vi "PerformScan.vi"(0 "Avg Num Mod":i32=1, 1 "Therapy/AVG ?":bool, 2 "AlazarCluster":T9, 5 "Line Axis":i32=1 min=1 max=4, 7 "Type of scan":T10, 9 "lines per scan plane mod":i32=128, 11 "Reverse ?":bool, 12 "Digitizer Settings":T5={"Digitizer delay (us) "=0.0, "rf points per line"=2048, "lines per plane"=128, "Samp Rate (Hz)"=100000000.0, "Additional dig delay (us)"=0.0, "Voltage Scale"=0.4, "Pre-Looks"=0, "Offset delay (us)"=0.0, "bits A/D"=8, "Avg Num"=1, "DigTimeOut"=5.0, "Rel Dig Delay"=0.0, "Dig Ch"=0, "LeCroyCluster"={"LeCroy Channels"=[TRUE, FALSE, FALSE, FALSE], "LC read pt offset"=0.0, "Sweep Avg"=FALSE}, "Main Digitizer"=enum."NI Digitizer", "Dig Config"=enum."Single channel", "Digitizer ID Cluster"={"Acqiris/Alazar/SP ID"=[], "NI Instr Handles"=[], "LeCroy VISA"="", "GaGe Handle"={"Handle"=0, "Sample size"=0, "Resolution"=0, "Offset"=0, "Channels"=0, "Boards"=0}, "ATS Ref"="ATS9350", "Acqiris Address"=["PCI::INSTR0"], "ADQRef"=refnum, "adq_cu_ptr"=refnum}, "Trigger Settings"={"Trig Source"=1, "Trig Coupling"=0, "Trig Slope"=0, "Level (mV)"=1500.0}, "Bulk Acq"=FALSE, "Bulk Start Indexes"=[], "Data Ref RF"=refnum, "NI ID/Channel"=[], "Total Dig CH"=1, "Xtra Ann Trig delay (us)"=10.0, "Fix Z Delay?"=FALSE, "One Way Transmission?"=FALSE, "Data Ref Log"=refnum} {"Trigger Settings"."Trig Slope" items=["Positive", "Negative"]; "Trigger Settings"."Level (mV)" format="%.2f"; "Trigger Settings"."Trig Coupling" items=["DC 1 MOhm", "AC 1 MOhm", "DC 50 Ohm", "AC 50 Ohm"]; "Trigger Settings"."Trig Source" items=["Chan 1", "External"]; "Rel Dig Delay" format="%.2f"; "DigTimeOut" format="%.2f"; "Avg Num" min=1; "Offset delay (us)" format="%.2f"; "Additional dig delay (us)" format="%.2f"; "Digitizer delay (us)" format="%.2f"}, 13 "Motion Settings In":T1={"No Motion?"=FALSE, "Motion System"=enum."NI 735x", "Motion Bd ID"=1, "Motion Profile"="SMAC1", "# Axis"=1, "Reverse Z axis?"=TRUE, "SMAC Axis"=0, "scan pair"=enum."y-(x) scan", "RT fps"=6.0, "Steps per mm"=[1000, 1000, 1000, 1000], "Motor Parameters"={"velocity ct/s"=[10000.0, 10000.0, 10000.0, 50000.0], "accel ct/s^2"=[50000.0, 50000.0, 50000.0, 200000.0]}, "One Way Scan"=FALSE, "Reverse One Way Scan"=FALSE, "Global Position (mm)"=[], "Plane"=0, "Distance between\nscan lines (um)"=0.0, "Distance between\nscan planes (um)"=0.0, "number of scan planes"=1, "Total steps in line"=0, "Xtra plane\ndistance  (um)"=100, "Xtra planes "=1, "Add Axis"=FALSE, "overshoot cts"=200, "BKPT Shift"=0, "Scan Start Time (ms)"=0, "ESP VISA"="GPIB::1::INSTR", "3rd Axis"=1, "GL Ref Out"=refnum, "Galil Address"=""} {"3rd Axis" items=["x", "y", "z", "w"]; "Xtra planes" min=1; "Xtra plane\ndistance  (um)" min=0; "Distance between\nscan planes (um)" format="%.2f"; "Distance between\nscan lines (um)" format="%.2f"; "SMAC Axis" items=["None"=0, "Axis 1"=1, "Axis 2"=2, "Axis 3"=3, "Axis 4"=4, "Axis 5"=5, "Axis 6"=6, "Axis 7"=7, "Axis 8"=8, "Vector Space 1"=17, "Vector Space 2"=18, "Vector Space 3"=19, "Vector Space 4"=20]; "Motion Bd ID" min=1 max=32 step=1}, 14 "File Names":string[](array[string]), 15 "Offset":dbl format="%.2f") -> ()   [LabVIEW 2022 SP3]
uses:
  -ScanSystem/Controls/ScanType2.ctl
  Digitizers/-DigitizerRoutines/DigitizerSettings.ctl
  Digitizers/-DigitizerRoutines/Digitizer.ctl
  Digitizers/-DigitizerRoutines/DigConfig.ctl
  Digitizers/-DigitizerRoutines/DigitizerID.ctl
  C:/Windows/System32/ADQAPI_dotNet_helper.dll
  MotionParameters.ctl
  MotionSys.ctl
  -MotionRoutines/ScanAxis.ctl
  -MotionRoutines/3rdAxis.ctl
  Galil/Command Menu.ctl
  <vilib>/Motion/FlexMotion/CustomControls/CustomControls.llb/Program.flx
panel:
  # "allows movement down axis where pulse is sent out every time Step to Move has\nbeen moved. Small program is sent to MM2000 and executed. Motion is kind of slow."
  # "1-D and 2-D B scan settings"
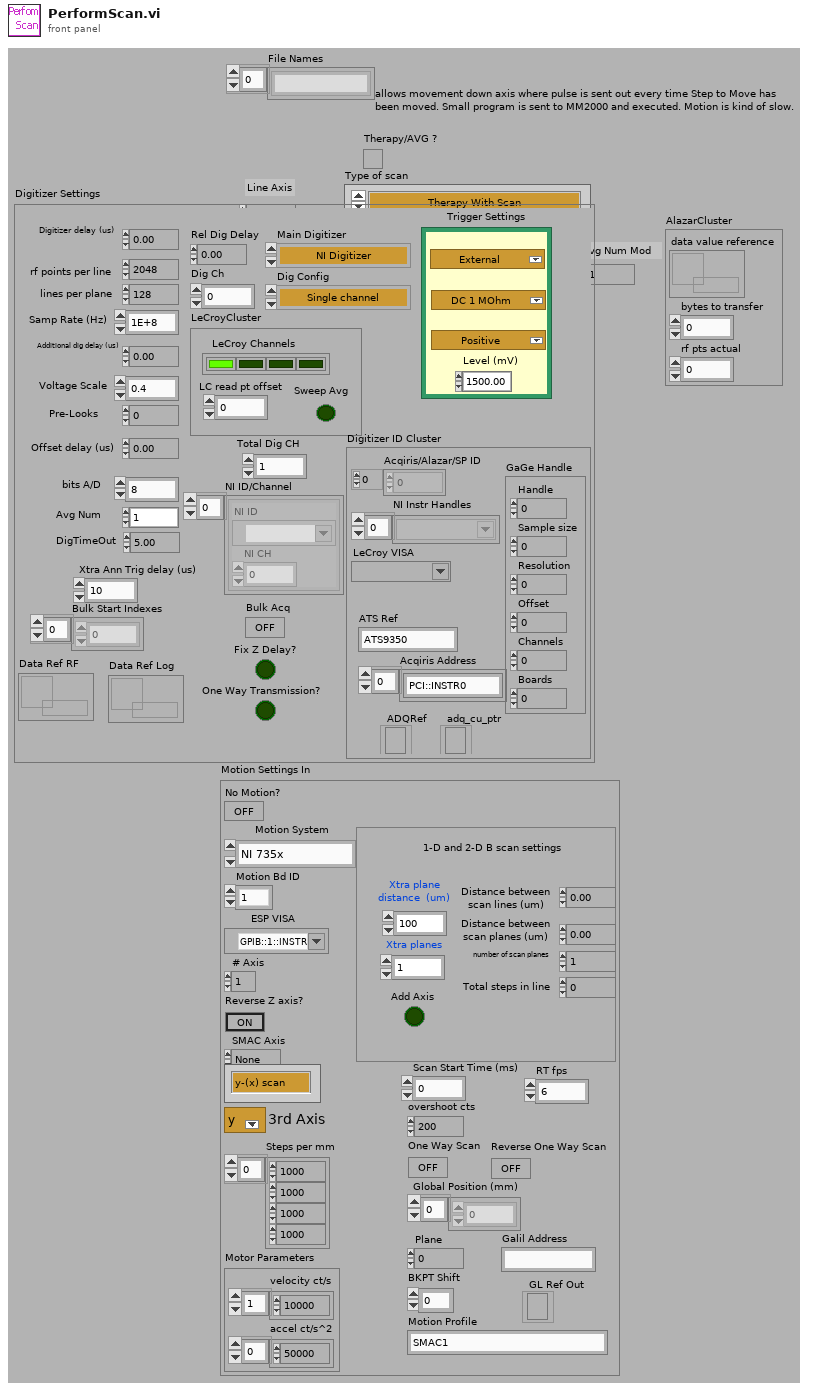
[diagram p1: front panel]
types:
  T1 = typedef "MotionParameters.ctl" = cluster{"No Motion?":bool, "Motion System":T2, "Motion Bd ID":u8, "Motion Profile":string, "# Axis":i8, "Reverse Z axis?":bool, "SMAC Axis":u16, "scan pair":T3, "RT fps":sgl, "Steps per mm":i32[], "Motor Parameters":cluster{"velocity ct/s":dbl[], "accel ct/s^2":dbl[]}, "One Way Scan":bool, "Reverse One Way Scan":bool, "Global Position (mm)":dbl[], "Plane":i32, "Distance between\nscan lines (um)":sgl, "Distance between\nscan planes (um)":sgl, "number of scan planes":i32, "Total steps in line":i32, "Xtra plane\ndistance  (um)":i32, "Xtra planes ":i32, "Add Axis":bool, "overshoot cts":i32, "BKPT Shift":i32, "Scan Start Time (ms)":u32, "ESP VISA":refnum<visa-resource-name>, "3rd Axis":T4, "GL Ref Out":refnum<k7>, "Galil Address":string}
  T2 = typedef "MotionSys.ctl" = enum16{"MM3000", "NI 735x", "Newport ESP", "No Motion Card", "Galil"}
  T3 = typedef "ScanAxis.ctl" = enum16{"y-(x) scan", "x-(y) scan", "z-(x) scan", "z-(y) scan", "y-(z) scan", "x-(z) scan", "w-(x) scan", "w-(y) scan", "w-(z) scan", "x-(w) scan", "y-(w) scan", "z-(w) scan"}
  T4 = typedef "3rdAxis.ctl" = u16
  T5 = typedef "DigitizerSettings.ctl" = cluster{"Digitizer delay (us) ":dbl, "rf points per line":i32, "lines per plane":i32, "Samp Rate (Hz)":dbl, "Additional dig delay (us)":dbl, "Voltage Scale":dbl, "Pre-Looks":i32, "Offset delay (us)":dbl, "bits A/D":i8, "Avg Num":i32, "DigTimeOut":sgl, "Rel Dig Delay":sgl, "Dig Ch":i32, "LeCroyCluster":cluster{"LeCroy Channels":bool[], "LC read pt offset":dbl, "Sweep Avg":bool}, "Main Digitizer":T6, "Dig Config":T7, "Digitizer ID Cluster":T8, "Trigger Settings":cluster{"Trig Source":u16, "Trig Coupling":u16, "Trig Slope":u16, "Level (mV)":dbl}, "Bulk Acq":bool, "Bulk Start Indexes":i32[], "Data Ref RF":refnum<data-value>, "NI ID/Channel":cluster{"NI ID":refnum<k15>, "NI CH":i32}[], "Total Dig CH":i32, "Xtra Ann Trig delay (us)":dbl, "Fix Z Delay?":bool, "One Way Transmission?":bool, "Data Ref Log":refnum<data-value>}
  T6 = typedef "Digitizer.ctl" = enum16{"Acqiris Digitizer", "NI Digitizer", "LeCroy", "GaGe", "AlazarTech", "No Digitizer", "Teledyne"}
  T7 = typedef "DigConfig.ctl" = enum16{"Single channel", "2 Chans w/ 2 Acqiris", "2 Chans w/ 1 Acqiris", "5-CH Pulser New", "5-CH pulser w/ ann array", "5-pass style ann array", "Empty"}
  T8 = typedef "DigitizerID.ctl" = cluster{"Acqiris/Alazar/SP ID":u32[], "NI Instr Handles":refnum<k15>[], "LeCroy VISA":refnum<visa-resource-name>, "GaGe Handle":cluster{"Handle":u32, "Sample size":u32, "Resolution":i32, "Offset":i32, "Channels":u32, "Boards":u32}, "ATS Ref":string, "Acqiris Address":string[], "ADQRef":refnum<k24>, "adq_cu_ptr":refnum<k24>}
  T9 = cluster{"data value reference":refnum<data-value>, "bytes to transfer":u32, "rf pts actual":u32}
  T10 = typedef "ScanType2.ctl" = enum16{"Therapy With Scan", "M scan", "M Scan With Therapy Burst", "1-D B Scan", "1-D B Scan With Therapy Burst", "2-D B Scan", "2-D B Scan With Therapy Burst", "Rotational Scan", "1-D B-Scan PRF", "2-D B-Scan PRF", "Real-Time Scan", "Contrast Agents", "1-D w/ Real-Time Set Up", "Dual Transducer", "Acoustic Microscopy", "Hydrophone Scanning"}
  T11 = typedef "Program.flx" = u8
  T12 = enum16{"Run/Stop", "Motor Off", "Velocity Threshold", "Move Complete"}
  T13 = typedef "Command Menu.ctl" = enum16{"CommandPassThrough", "Abort Motion", "Define Pos", "Velocity", "Acceleration", "Deceleration", "Position Rel", "Postion Abs", "Begin Move", "After Move", "Home", "KI", "KD", "KP", "IL", "Config I/O", "Set Bit", "Clear Bit", "Motor Off", "Moto On", "Status", "Execute", "Halt Execute", "HX Status", "Tell Velocity", "Check Motion", "BreakPoint", "Tell Position", "Current Code Line", "Tell Switches", "OC Force On", "OC Off", "Pos Soft Limit", "Rev Soft Limit"}
  T14 = typedef "Bd Id Out" = u8
  T15 = typedef "Resource Out (Enum).flx" = u16
  T16 = typedef "Axis Status (8 axes).flx" = cluster{"1":bool, "2":bool, "3":bool, "4":bool, "5":bool, "6":bool, "7":bool, "8":bool}
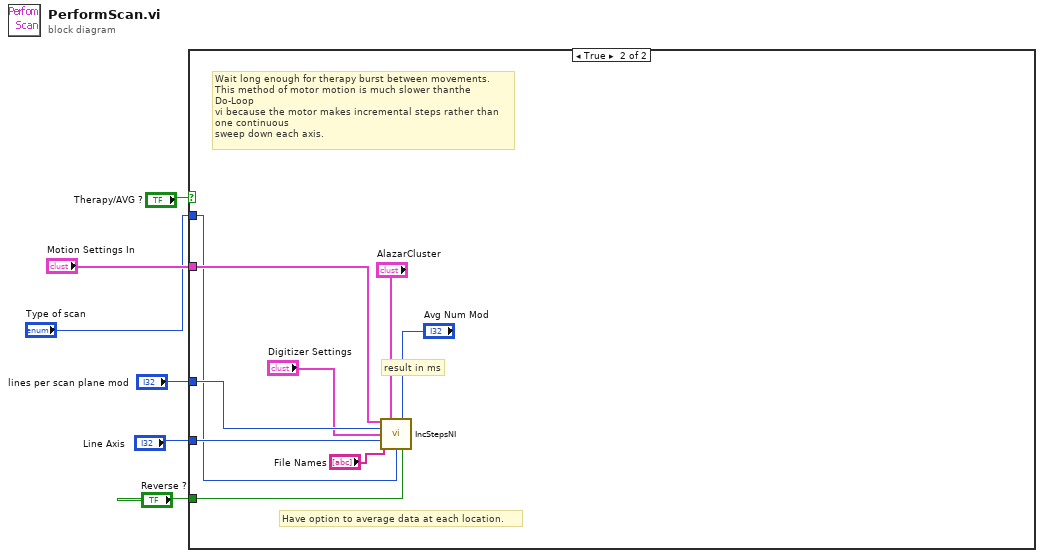
[diagram p0: block diagram]
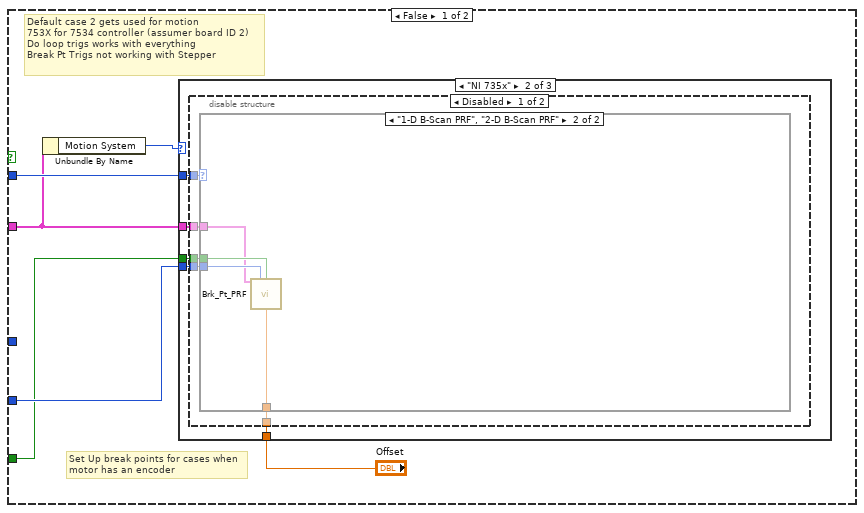
[diagram p2: hidden frame]
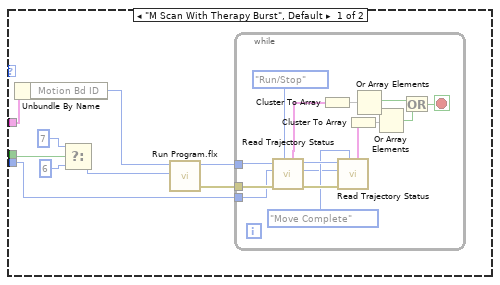
[diagram p4: hidden frame]
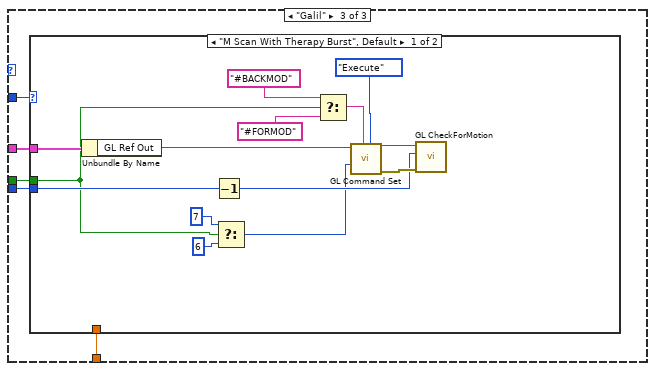
[diagram p6: hidden frame]
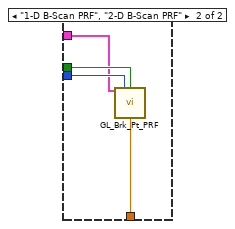
[diagram p7: hidden frame]
diagram:
  n1 = case shown="True" "Therapy/AVG ?" {
    tunnel: "Line Axis" -> [w12 w82]
    tunnel: "lines per scan plane mod" -> [_ w81]
    tunnel: "Reverse ?" -> [w11 w80]
    tunnel: "Motion Settings In" -> [w8 w75]
    tunnel: "Type of scan" -> [w9 w74]
    frame False {
      # "Default case 2 gets used for motion\n753X for 7534 controller (assumer board ID 2)\nDo loop trigs works with everything\nBreak Pt Trigs not working with Stepper"
      # "Set Up break points for cases when motor has an encoder"
      n2 = Unbundle By Name(w8) -> ("Motion System"=w7:T2)
      n3 = case shown="\"NI 735x\"" w7 {
        tunnel: w12 -> [_ w17 w55]
        tunnel: w11 -> [_ w16 w54]
        tunnel: "Offset" -> [_ w15 w53]
        tunnel: w8 -> [_ w14 w52]
        tunnel: w9 -> [_ w13 w51]
        frame "MM3000", Default {
        }
        frame "NI 735x" {
          n4 = disable-structure shown="Disabled" {
            disable-tunnel: w17 -> [w22 _]
            disable-tunnel: w16 -> [w21 _]
            disable-tunnel: w15 -> [w20 _]
            disable-tunnel: w14 -> [w19 _]
            disable-tunnel: w13 -> [w18 _]
            frame Disabled {
              n5 = case shown="\"1-D B-Scan PRF\", \"2-D B-Scan PRF\"" w18 {
                tunnel: w22 -> [w23 w50]
                tunnel: w21 -> [w30 w49]
                tunnel: w20 -> [_ w48]
                tunnel: w19 -> [w27 w47]
                frame "M Scan With Therapy Burst", Default {
                  n6 = Unbundle By Name(w27) -> ("Motion Bd ID"=w26:u8)
                  n7 = Select(t=T11 7 ("Program (1)"), s=w30, f=T11 6 ("Program (1)")) -> (s? t:f=w31:T11)
                  n8 = call <vilib>:"Run Program.flx"("Program (1)"=w31, "Board ID"=w26) -> ("error out"=w24:errorcluster, "Bd ID Out"=w25:T14)  [unwired: 1 in, 4 out]
                  n9 = while {
                    tunnel: w25 -> [w46]
                    tunnel: w24 -> [w42]
                    tunnel: w23 -> [w33]
                    stop <- w34 stop-if-true
                    n10 = call <vilib>:"Read Trajectory Status.vi"("Status Type"=T12."Run/Stop", "error in (no error)"=w42, "Axis or Vector Space"=w33, "Board ID"=w46) -> ("error out"=w40:errorcluster, "Resource Output"=w32:T15, "Bd ID Out"=w41:T14, "Status"=w44:T16)  [unwired: 2 in]
                    n11 = Cluster To Array(cluster=w44) -> (array=w43:bool[])
                    n12 = call <vilib>:"Read Trajectory Status.vi"("Status Type"=T12."Move Complete", "error in (no error)"=w40, "Axis or Vector Space"=w32, "Board ID"=w41) -> ("Status"=w39:T16)  [unwired: 2 in, 3 out]
                    n13 = Cluster To Array(cluster=w39) -> (array=w37:bool[])
                    n14 = Or Array Elements(Boolean array=w43) -> (logical OR=w36:bool)
                    n15 = Or Array Elements(Boolean array=w37) -> (logical OR=w35:bool)
                    n16 = Or(x=w36, y=w35) -> (x .or. y?=w34:bool)
                  }
                }
                frame "1-D B-Scan PRF", "2-D B-Scan PRF" {
                  n17 = call "Brk_Pt_PRF.vi"("Motion Settings In"=w47, "Axis"=w50, "Reverse ?"=w49, "Offset"=w48) -> ()  [unwired: 4 in, 8 out]
                }
              }
            }
            frame Enabled {
            }
          }
        }
        frame "Galil" {
          n18 = case shown="\"M Scan With Therapy Burst\", Default" w51 {
            tunnel: w55 -> [w60 w73]
            tunnel: w54 -> [w57 w72]
            tunnel: w53 -> [_ w71]
            tunnel: w52 -> [w69 w70]
            frame "M Scan With Therapy Burst", Default {
              n19 = Unbundle By Name(w69) -> ("GL Ref Out"=w64:refnum<k7>)
              n20 = Decrement(x=w60) -> (x-1=w61:i32)
              n21 = Select(t=u8 7 ("Program (1)"), s=w57, f=u8 6 ("Program (1)")) -> (s? t:f=w56:u8)
              n22 = Select(t="#BACKMOD" ("Program Name"), s=w57, f="#FORMOD" ("Program Name")) -> (s? t:f=w65:string)
              n23 = call "GL Command Set.vi"("Command"=Command_Menu."Execute", "Text Input"=w65, "Value"=w56, "Galil.IGalil"=w64) -> ("error out"=w62:errorcluster, "ref out"=w63:refnum<k7>)  [unwired: 3 in, 3 out]
              n24 = call "GL CheckForMotion.vi"("error in"=w62, "Axis"=w61, "Refnum in"=w63) -> ()  [unwired: 6 in, 3 out]
            }
            frame "1-D B-Scan PRF", "2-D B-Scan PRF" {
              n25 = call "GL_Brk_Pt_PRF.vi"("Motion Settings In"=w70, "Axis"=w73, "Reverse ?"=w72, "Offset"=w71) -> ()  [unwired: 7 in, 5 out]
            }
          }
        }
      }
    }
    frame True {
      # "Have option to average data at each location."
      # "Wait long enough for therapy burst between movements.\nThis method of motor motion is much slower thanthe Do-Loop\nvi because the motor makes incremental steps rather than one continuous\nsweep down each axis."
      # "result in ms"
      n26 = call "IncStepsNI.vi"("Motion Settings In"=w75, "AlazarCluster"="AlazarCluster", "Avg Num"="Avg Num Mod", "scans lines"=w81, "Digitizer Settings"="Digitizer Settings", "Axis"=w82, "File Names"="File Names", "Type of scan"=w74, "Reverse ?"=w80) -> ()  [unwired: 2 in, 5 out]
    }
  }
